vi "StrIpToByteArr.vi"(1 "CANET IP":string) -> (0 "Array":u8[](array[numeric]))   [LabVIEW 2014]
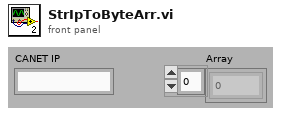
[diagram p1: front panel]
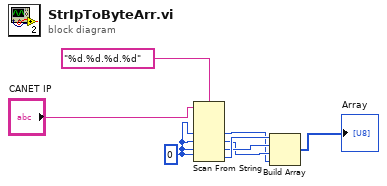
[diagram p0: block diagram]
diagram:
  w8 = u8 0 ("default value 4")
  n1 = Scan From String(format string="%d.%d.%d.%d", input string="CANET IP", default 1=w8, default 2=w8, default 3=w8, default 4=w8) -> (output 1=w2:u8, output 2=w3:u8, output 3=w4:u8, output 4=w5:u8)  [unwired: 2 in, 3 out]
  n2 = Build Array(w5, w4, w3, w2) -> (→"Array":u8[])
